vi "Clase220222.vi"() -> ()   [LabVIEW 2021]
panel:
  in  "Enum":T1(ring)
  in  "b":dbl
  in  "a":dbl
  out "c":dbl
  in  "stop":bool
  # "Mendoza Meza Manuel Everardo"
  # "0-9. -\n10-19. +\n20-29. *\n30-39. /"
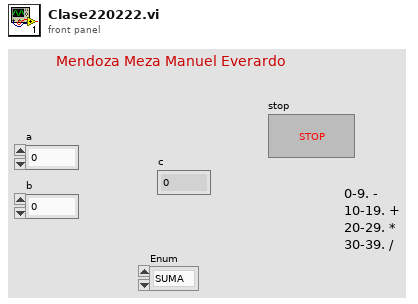
[diagram p1: front panel]
types:
  T1 = enum16{"SUMA", "RESTA", "MULTIPLICACION", "DIVISION"}
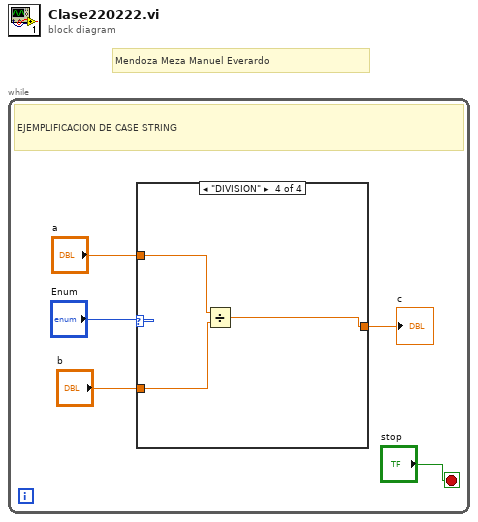
[diagram p0: block diagram]
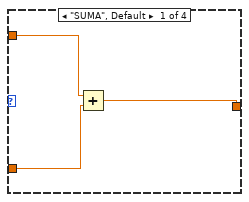
[diagram p2: hidden frame]
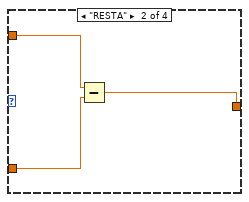
[diagram p3: hidden frame]
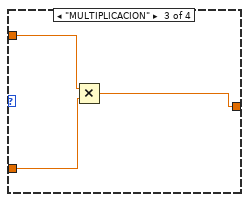
[diagram p4: hidden frame]
diagram:
  # "Mendoza Meza Manuel Everardo"
  n1 = while {
    stop <- "stop" stop-if-true
    # "EJEMPLIFICACION DE CASE STRING"
    n2 = case shown="\"DIVISION\"" "Enum" {
      tunnel: [w6 w9 w12 w15] -> w3
      tunnel: "b" -> [w7 w10 w13 w16]
      tunnel: "a" -> [w8 w11 w14 w17]
      frame "SUMA", Default {
        n3 = Add(x=w8, y=w7) -> (x+y=w6:dbl)
      }
      frame "RESTA" {
        n4 = Subtract(x=w11, y=w10) -> (x-y=w9:dbl)
      }
      frame "MULTIPLICACION" {
        n5 = Multiply(x=w14, y=w13) -> (x*y=w12:dbl)
      }
      frame "DIVISION" {
        n6 = Divide(x=w17, y=w16) -> (x/y=w15:dbl)
      }
    }
    "c" <- w3
  }
